vi "LP_Help.vi"   [LabVIEW 2012]
uses:
  SubVIs/LVPresent_Globals.vi
panel:
  # "If you need to go back more than a slide at a time, press the up arrow to see the entire presentation."
  # "Need Help?\n\nIf you ever need help at any point, click on the help button in the bottom left corner of the screen. It should address any questions you have throughout the tutorial. Also, I would recommend pulling up the context help while you code to provide additional help (Help-->Show Context Help). It wouldn't be a bad idea to take a peek at the help menu now just for reference.\n\n\nNow that we've checked out the board, lets take a look at the coding."
  # "This button ends the presentation, and takes you back to the selector screen!"
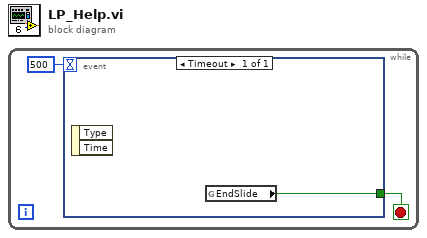
[diagram p0: block diagram]
diagram:
  n1 = while {
    stop <- w2 stop-if-true
    n2 = event shown="[0] Timeout" {
      selector: _ -> [_]
      dyn-events: _ -> [_]
      timeout: 500 -> [_]
      tunnel: [w3] -> w2
      event Timeout {
        n3 = event-data() -> ()  [unwired: 1 in, 2 out]
        n4 = global read "LVPresent_Globals.vi" "EndSlide"() -> (w3:bool)
      }
    }
  }
